vi "Mix Coordinates Array.vi"(8 "I_Required Length":i32, 9 "I_Number of columns":i16, 11 "I_Number of rows":i16) -> (1 "O_Mixed RGB Coordinates":i32[](array[numeric]), 3 "O_Mixed Coordinates":i32[][](array[numeric]))   [LabVIEW 2015]
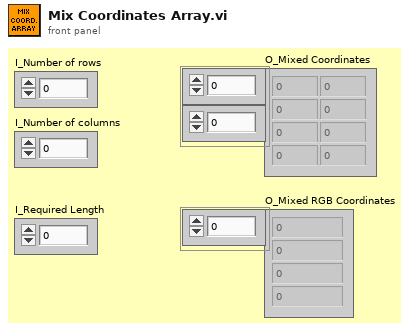
[diagram p1: front panel]
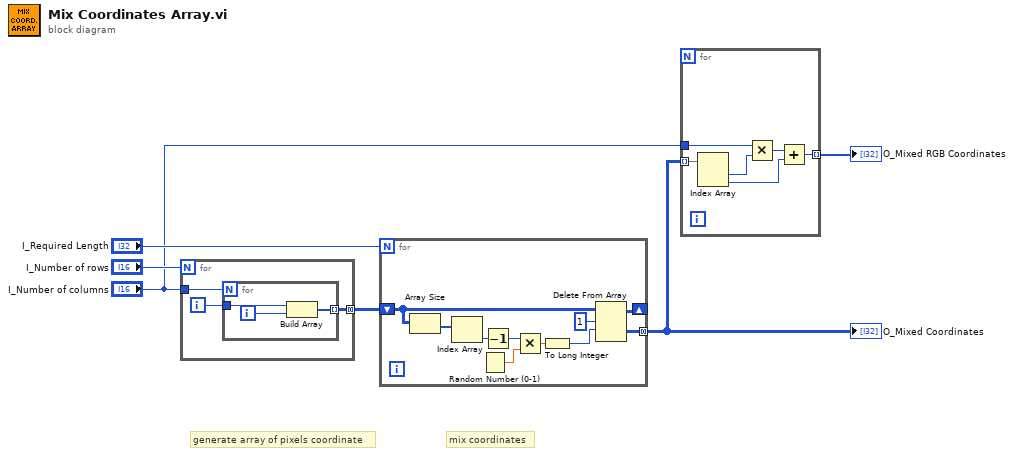
[diagram p0: block diagram]
diagram:
  # "mix coordinates"
  # "generate array of pixels coordinate"
  n1 = for {
    N: "I_Number of rows" -> [_]
    tunnel: [w8] -> w6 mode=concatenating
    tunnel: "I_Number of columns" -> [w9]
    i -> [w7]
    n2 = for {
      N: w9 -> [_]
      tunnel: [w12] -> w8 mode=indexing
      tunnel: w7 -> [w11]
      i -> [w10]
      n3 = Build Array(w11, w10) -> (w12:i32[])
    }
  }
  n4 = for {
    N: "I_Required Length" -> [_]
    shift-right: [w20] -> _
    shift-left: w6 -> [w19]
    tunnel: [w21] -> w3 mode=concatenating
    n5 = Array Size(array=w19) -> (size(s)=w14:i32[])
    n6 = Index Array(array=w14) -> (element=w13:i32)  [unwired: 1 in]
    n7 = Random Number (0-1)() -> (number: 0 to 1=w18:dbl)
    n8 = Decrement(x=w13) -> (x-1=w16:i32)
    n9 = Multiply(x=w16, y=w18) -> (x*y=w17:dbl)
    n10 = To Long Integer(number=w17) -> (32bit integer=w15:i32)
    n11 = Delete From Array(array=w19, length=1, index (row)=w15) -> (deleted portion=w21:i32[][], array with subset deleted=w20:i32[][])  [unwired: 1 in]
  }
  "O_Mixed Coordinates" <- w3
  n12 = for {
    tunnel: w3 -> [w28] mode=indexing
    tunnel: "I_Number of columns" -> [w26]
    tunnel: [w23] -> w1 mode=indexing
    n13 = Index Array(array=w28) -> (element #1=w27:i32, element #2=w24:i32)  [unwired: 2 in]
    n14 = Multiply(x=w26, y=w27) -> (x*y=w25:i32)
    n15 = Add(x=w25, y=w24) -> (x+y=w23:i32)
  }
  "O_Mixed RGB Coordinates" <- w1
